vi "example_VL Receive.vi"(10 "port":u32=1, 11 "board":u32) -> (0 "error out":errorcluster)   [LabVIEW 2020]
uses:
  src/_controls/comm_computedMAC-IP.ctl
  src/_controls/comm_verification_rx.ctl
  src/_controls/comm_udp_rx.ctl
  <extravilib>/ChannelInstances/Tag-bool/Write With Abort.vi
  <extravilib>/ChannelInstances/Tag-bool/Read With Abort.vi
  src/_polimorphicInstances/session/CreateSession(Rx-VL-Oriented).vi
  src/bsp/AFDX_Receive/Create Rx VL.vi
  src/_polimorphicInstances/udpPort/CreateUdpPort(RX-CommPort).vi
  src/_polimorphicInstances/control/Start (Rx).vi
  <extravilib>/ChannelInstances/Tag-bool/Instantiate.vi
  <extravilib>/ChannelInstances/Tag-bool/EndpointRead.vi
  <extravilib>/ChannelInstances/Tag-bool/Endpoint.vi
  src/_polimorphicInstances/control/Stop (Rx).vi
  src/AIM664LV.lvlib
  <extravilib>/ChannelInstances/Tag-bool.lvlib
panel:
  out "errCount":u32[](array[numeric])
  out "MsgCount":u32[](array[numeric])
  out "current time":timestamp=timestamp(3686488955.9671674 s since 1904-01-01)
  in  "Tab Control":enum32{"Configuration", "Status"}(tab)
  in  "DefaultPayloadMode (Full)":u32(ring) items=["FDX_PAYLOAD_FULL", "FDX_PAYLOAD_IP_EXT", "FDX_PAYLOAD_IP", "FDX_PAYLOAD_MAC"]
  out "CommPort Addresses":T1[](array[typedef])=[{"MACsrc"=[], "IPsrc"="10.1.33.1", "IPdest"="224.224.0.60"}, {"MACsrc"=[], "IPsrc"="10.1.33.1", "IPdest"="224.224.0.60"}] {"MACsrc" format="%.0x"}
  in  "VL Config":T2={"VlId"=60, "VLRange"=2, "VerificationMode"=0, "Bag"=0, "Jitter"=0, "MaxFrameLength"=0, "MaxSkew"=0, "VLBufSize"=32768, "FilterMode"=0, "FilterPosition"=0, "Padding"=0, "FilterMask"=0, "FilterData"=0, "MinFrameLength"=0} {"FilterMode" items=["FDX_RX_VL_FLT_DIS", "FDX_RX_VL_FLT_ENA ", "FDX_RX_VL_FLT_ENA_INV"]; "MaxFrameLength" format="%.0x"; "VerificationMode" items=["FDX_RX_VL_CHECK_ENA_DEFAULT"=65535, "FDX_RX_VL_CHECK_REDMAM"=16, "DX_RX_VL_CHECK_TRAFIC"=8, "FDX_RX_VL_CHECK_FRAMESIZE"=4, "FDX_RX_VL_CHECK_SNINTEG"=2, "FDX_RX_VL_CHECK_INVPAC"=1, "FDX_RX_VL_CHECK_DISA"=0]}
  in  "CommPort Config":T3[](array[typedef])=[{"PortType"=enum."FDX_UDP_SAMPLING", "SubVIId"=1, "domainID"=1, "sideID"=1, "locationID"=1, "partitionID"=1, "UdpSrcPort"=1, "UdpDstPort"=1, "UdpNumBufMessages"=1, "UdpMaxMessageSize"=1000, "UdpSamplingRate"=0}, {"PortType"=enum."FDX_UDP_SAMPLING", "SubVIId"=2, "domainID"=1, "sideID"=1, "locationID"=1, "partitionID"=1, "UdpSrcPort"=2, "UdpDstPort"=2, "UdpNumBufMessages"=1, "UdpMaxMessageSize"=1000, "UdpSamplingRate"=0}] {"partitionID" format="%.0b"}
  out "BytesRead":u32[](array[numeric])
  out "read time uS":u32(graph)=3177
  in  "poll rate mS 1":u32=10
  out "data":cluster{"Data":u8[]}[](array[cluster])
  out "current irig time":T4
  in  "stop":bool
  out "PortInitOut":T5 {"PortConfig" items=["FDX_SINGLE", "FDX_REDUNDANT"]}
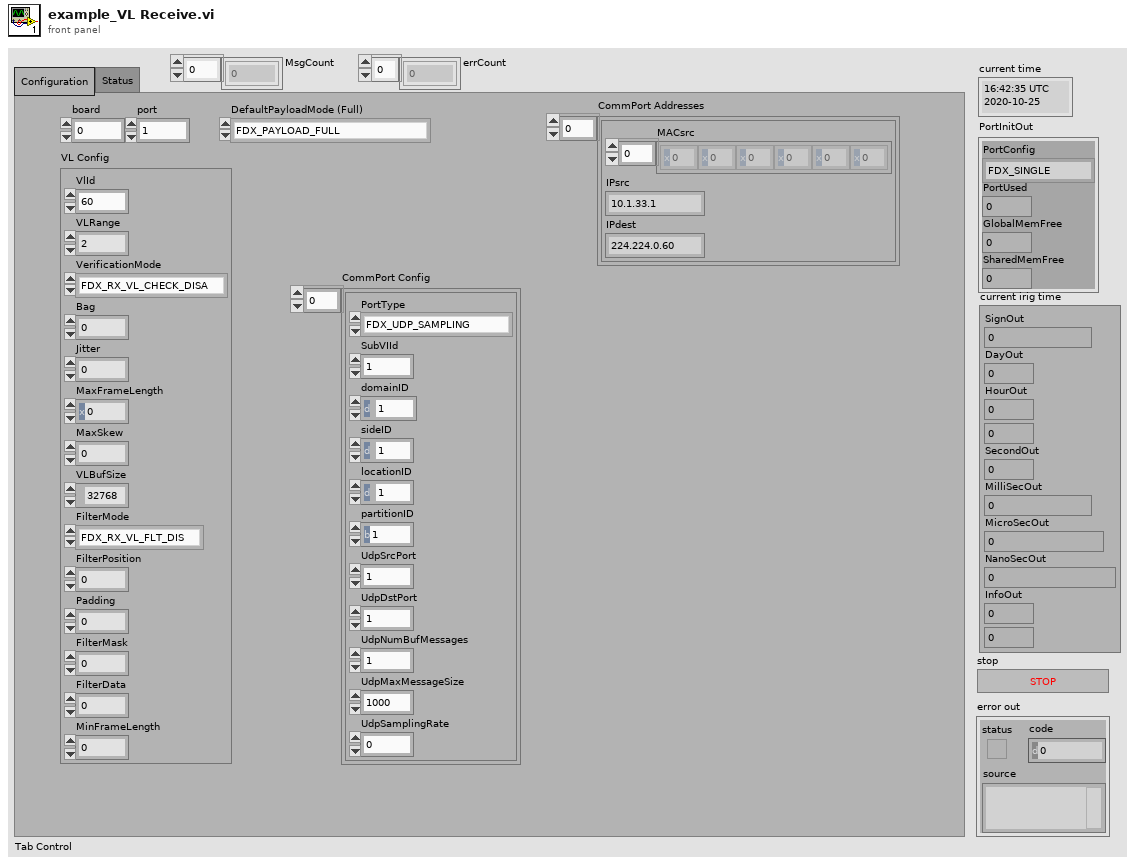
[diagram p1: front panel]
types:
  T1 = typedef "AIM664LV.lvlib/comm_computedMAC-IP.ctl" = cluster{"MACsrc":u8[], "IPsrc":string, "IPdest":string}
  T2 = typedef "AIM664LV.lvlib/comm_verification_rx.ctl" = cluster{"VlId":u16, "VLRange":u32, "VerificationMode":u32, "Bag":u32, "Jitter":u32, "MaxFrameLength":u32, "MaxSkew":u32, "VLBufSize":u32, "FilterMode":u32, "FilterPosition":u32, "Padding":u32, "FilterMask":u32, "FilterData":u32, "MinFrameLength":u32}
  T3 = typedef "AIM664LV.lvlib/comm_udp_rx.ctl" = cluster{"PortType":enum16{"FDX_UDP_SAMPLING", "FDX_UDP_QUEUING"}, "SubVIId":u32, "domainID":u8, "sideID":u8, "locationID":u8, "partitionID":u8, "UdpSrcPort":u16, "UdpDstPort":u16, "UdpNumBufMessages":u32, "UdpMaxMessageSize":u32, "UdpSamplingRate":u32}
  T4 = cluster{"SignOut":i32, "DayOut":u32, "HourOut":u32, "MinOut":u32, "SecondOut":u32, "MilliSecOut":u32, "MicroSecOut":u32, "NanoSecOut":u32, "InfoOut":u32, "Mode":u32}
  T5 = cluster{"PortConfig":u32, "PortUsed":u32, "GlobalMemFree":u32, "SharedMemFree":u32}
  T6 = typedef "Tag-bool.lvlib/))Channel.ctl" = refnum<queue>
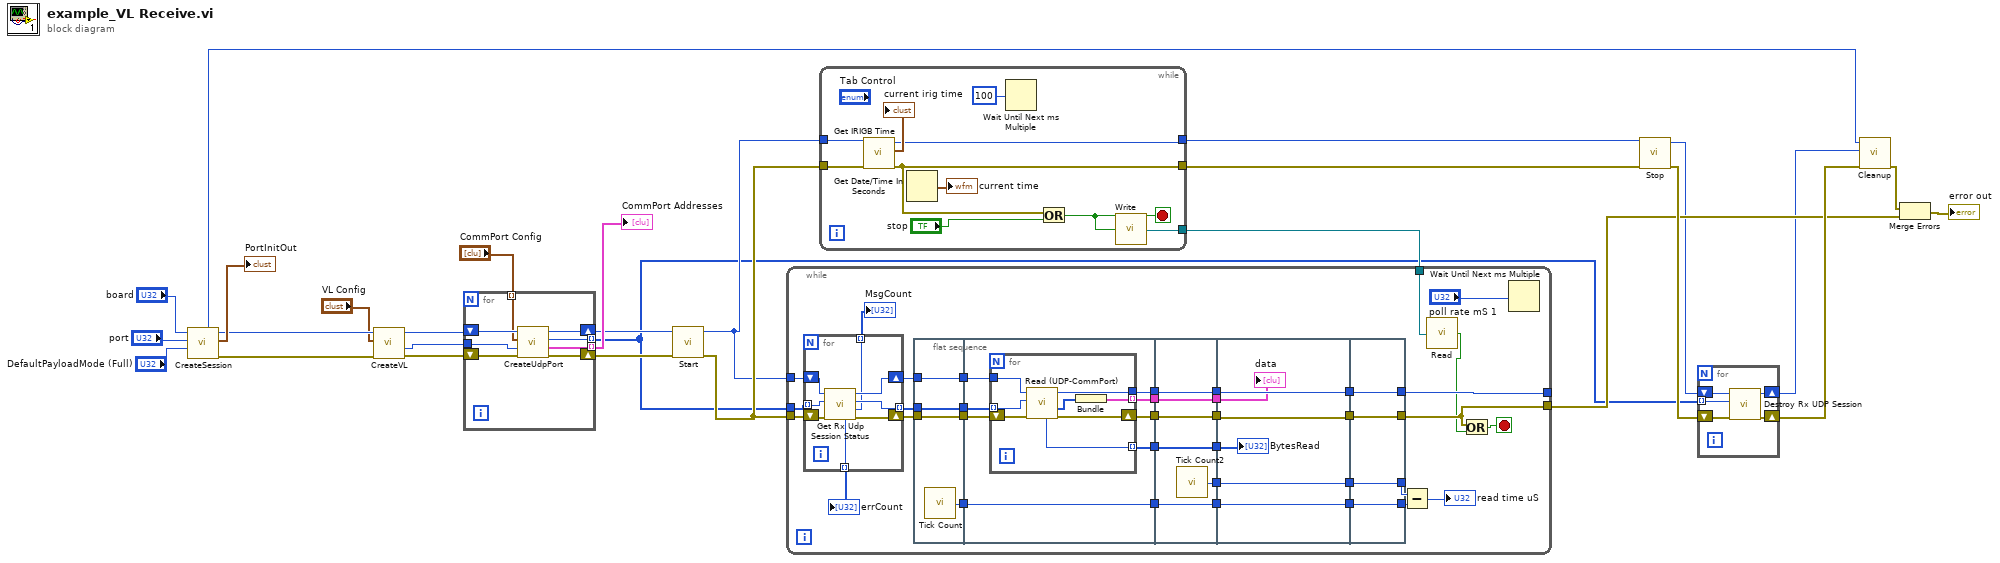
[diagram p0: block diagram]
diagram:
  n1 = call-poly "CreateSession.vi"("DefaultPayloadMode (Full)"="DefaultPayloadMode (Full)", "port"="port", "board"="board") -> ("error out"=w12:errorcluster, "PortInitOut"=→"PortInitOut":T5, "InstrumentHandle_port out"=w13:u32, "InstrumentHandle_board out"=w1:u32)  [unwired: 3 in, 2 out]
  n2 = call-poly "CreateVL.vi"("error in (no error)"=w12, "VL Config"="VL Config", "InstrumentHandle_port in"=w13) -> ("error out"=w9:errorcluster, "VlId"=w8:u16, "InstrumentHandle_port out"=w10:u32)  [unwired: 6 in]
  n3 = for {
    tunnel: [w35] -> w27 mode=indexing
    tunnel: [w31] -> w2 mode=indexing
    shift-right: [w36] -> w28
    shift-left: w9 -> [w33]
    shift-right: [w34] -> w26
    shift-left: w10 -> [w32]
    tunnel: w8 -> [w30]
    tunnel: "CommPort Config" -> [w29] mode=indexing
    n4 = call-poly "CreateUdpPort.vi"("error in (no error)"=w33, "VlId"=w30, "CommPort Config"=w29, "port handle in"=w32) -> ("error out"=w36:errorcluster, "computedAddresses"=w35:T1, "commPort handle out"=w31:u32, "port handle out"=w34:u32)  [unwired: 4 in]
  }
  "CommPort Addresses" <- w27
  n5 = call-poly "Start.vi"("error in (no error)"=w28, "InstrumentHandle_port in"=w26) -> ("error out"=w19:errorcluster, "InstrumentHandle_port out"=w3:u32)  [unwired: 8 in]
  n6 = while {
    tunnel: w3 -> [w45]
    tunnel: w19 -> [w44]
    tunnel: [w42] -> w22
    tunnel: [w41] -> w21
    tunnel: [w37] -> w17
    stop <- w38 stop-if-true
    n7 = call "Get IRIGB Time.vi"("error in (no error)"=w44, "InstrumentHandle_board in"=w45) -> ("error out"=w41:errorcluster, "Curent Irig Time"=→"current irig time":T4, "InstrumentHandle_board out"=w42:u32)  [unwired: 7 in]
    n8 = Get Date/Time In Seconds() -> (seconds since 1Jan1904=→"current time":timestamp)
    n9 = Wait Until Next ms Multiple(millisecond multiple=u32 100) -> ()  [unwired: 1 out]
    n10 = Or(x=w41, y="stop") -> (x .or. y?=w38:bool)
    n11 = call <extravilib>:"Write.vi"("element"=w38) -> ("channel"=w37:T6)  [unwired: 1 out]
  }
  n12 = while {
    tunnel: w19 -> [w53]
    tunnel: w2 -> [w52]
    tunnel: [w70] -> _
    tunnel: [w63] -> w14
    tunnel: w17 -> [w58]
    tunnel: w3 -> [w54]
    stop <- w82 stop-if-true
    n13 = for {
      shift-right: [w89] -> w47
      shift-left: w53 -> [w90]
      tunnel: w52 -> [w87] mode=indexing
      shift-right: [w86] -> w51
      shift-left: w54 -> [w88]
      tunnel: [w85] -> w50 mode=indexing
      tunnel: [w84] -> w49 mode=indexing
      tunnel: [w83] -> w48 mode=indexing
      n14 = call "Get Rx Udp Session Status.vi"("error in (no error)"=w90, "UdpHandle in"=w87, "InstrumentHandle_port in"=w88) -> ("error out"=w89:errorcluster, "MsgCount"=w84:u32, "UdpHandle out"=w85:u32, "InstrumentHandle_port out"=w86:u32, "MsgErrorCount"=w83:u32)  [unwired: 4 in]
    }
    "MsgCount" <- w49
    "errCount" <- w48
    n15 = flat-sequence {
      tunnel: w47 -> [w93]
      tunnel: w50 -> [w94]
      tunnel: [w94] -> w78
      tunnel: [w93] -> w77
      tunnel: [w92] -> w76
      tunnel: w51 -> [w91]
      tunnel: [w91] -> w55
      tunnel: w78 -> [w96]
      tunnel: w77 -> [w102]
      tunnel: w76 -> [w101]
      tunnel: [w101] -> w75
      tunnel: [w100] -> w67
      tunnel: [w99] -> w64
      tunnel: [w98] -> w61
      tunnel: [w97] -> w59
      tunnel: w55 -> [w95]
      tunnel: w75 -> [w116]
      tunnel: [w116] -> w74
      tunnel: [w115] -> w71
      tunnel: [w114] -> w68
      tunnel: w67 -> [w114]
      tunnel: [w113] -> w65
      tunnel: w64 -> [w113]
      tunnel: [w112] -> w62
      tunnel: w61 -> [w112]
      tunnel: [w111] -> w60
      tunnel: w59 -> [w111]
      tunnel: w74 -> [w122]
      tunnel: [w122] -> w80
      tunnel: [w121] -> w72
      tunnel: w71 -> [w121]
      tunnel: [w120] -> w69
      tunnel: w68 -> [w120]
      tunnel: [w119] -> w66
      tunnel: w65 -> [w119]
      tunnel: w62 -> [w117]
      tunnel: w60 -> [w118]
      tunnel: [w126] -> w81
      tunnel: w80 -> [w126]
      tunnel: [w125] -> w73
      tunnel: w72 -> [w125]
      tunnel: [w124] -> w70
      tunnel: w69 -> [w124]
      tunnel: [w123] -> w63
      tunnel: w66 -> [w123]
      frame #0 {
        n16 = call "Tick Count"() -> ("Tick Count(uSec)"=w92:u32)
      }
      frame #1 {
        n17 = for {
          tunnel: [w109] -> w100
          tunnel: [w103] -> w98 mode=indexing
          tunnel: [w107] -> w97 mode=indexing
          tunnel: w96 -> [w106] mode=indexing
          tunnel: w95 -> [w105]
          shift-right: [w108] -> w99
          shift-left: w102 -> [w110]
          n18 = call "Read (UDP-CommPort).vi"("error in (no error)"=w110, "UdpHandle in"=w106, "InstrumentHandle_port in"=w105) -> ("error out"=w108:errorcluster, "Data"=w104:u8[], "InstrumentHandle_port out"=w109:u32, "MsgRead"=w107:u32)  [unwired: 4 in, 1 out]
          n19 = Bundle("Data"=w104) -> (w103:cluster{"Data":u8[]})  [unwired: 1 in]
        }
      }
      frame #2 {
        n20 = call "Tick Count2"() -> ("Tick Count(uSec)"=w115:u32)
      }
      frame #3 {
        "BytesRead" <- w118
        "data" <- w117
      }
      frame #4 {
      }
    }
    n21 = Subtract(x=w73, y=w81) -> (x-y=→"read time uS":u32)
    n22 = call <extravilib>:"Read.vi"("channel"=w58) -> ("element"=w57:bool)  [unwired: 1 in, 1 out]
    n23 = Or(x=w63, y=w57) -> (x .or. y?=w82:bool)
    n24 = Wait Until Next ms Multiple(millisecond multiple="poll rate mS 1") -> ()  [unwired: 1 out]
  }
  n25 = call-poly "Stop.vi"("error in (no error)"=w21, "InstrumentHandle_port in"=w22) -> ("error out"=w20:errorcluster, "InstrumentHandle_port out"=w5:u32)  [unwired: 8 in]
  n26 = for {
    tunnel: w2 -> [w127] mode=indexing
    shift-right: [w130] -> w18
    shift-left: w20 -> [w131]
    shift-right: [w128] -> w4
    shift-left: w5 -> [w129]
    n27 = call "Destroy Rx UDP Session.vi"("error in (no error)"=w131, "UdpHandle in"=w127, "InstrumentHandle_port in"=w129) -> ("error out"=w130:errorcluster, "InstrumentHandle_port out"=w128:u32)  [unwired: 7 in]
  }
  n28 = call "Cleanup.vi"("error in (no error)"=w18, "InstrumentHandle_port in"=w4, "InstrumentHandle_board in"=w1) -> ("error out"=w16:errorcluster)  [unwired: 8 in]
  n29 = Merge Errors(w16, w14) -> (→"error out":errorcluster)
